vi "LIN_HoldEOL.vi"(5 "log?":bool, 7 "NAD":u8 format="%.0x", 8 "Error In":errorcluster caption="错误输入", 10 "exit":refnum<vi>, 11 "LIN Device":T1={"Master Frame(3C)"="MasterReq\nSPA3414_ConfigurationsCMAGeely_CEMCALYPSOSDB34XX0Cfg_LIN3_190709_", "Slave Frame(3D)"="SlaveResp\nSPA3414_ConfigurationsCMAGeely_CEMCALYPSOSDB34XX0Cfg_LIN3_190709_", "Request Schedule"="CEMLIN3DiagRequestSchedule\nSPA3414_ConfigurationsCMAGeely_CEMCALYPSOSDB34XX0Cfg_LIN3_190709_", "Response Schedule"="CEMLIN3DiagResponseSchedule\nSPA3414_ConfigurationsCMAGeely_CEMCALYPSOSDB34XX0Cfg_LIN3_190709_", "Frame Write SCU"="", "Frame Read SCU"="", "LIN Name"=""}) -> (0 "error IO":errorcluster)   [LabVIEW 2018]
uses:
  Crl/LIN_DataType.ctl
  user VI's/LIN/LIN Device.ctl
panel:
  in  "y":u32=3000
  out "LIN Device":T1={"Master Frame(3C)"="MasterReq\nSPA3414_ConfigurationsCMAGeely_CEMCALYPSOSDB34XX0Cfg_LIN3_190709_", "Slave Frame(3D)"="SlaveResp\nSPA3414_ConfigurationsCMAGeely_CEMCALYPSOSDB34XX0Cfg_LIN3_190709_", "Request Schedule"="CEMLIN3DiagRequestSchedule\nSPA3414_ConfigurationsCMAGeely_CEMCALYPSOSDB34XX0Cfg_LIN3_190709_", "Response Schedule"="CEMLIN3DiagResponseSchedule\nSPA3414_ConfigurationsCMAGeely_CEMCALYPSOSDB34XX0Cfg_LIN3_190709_", "Frame Write SCU"="", "Frame Read SCU"="", "LIN Name"=""}
  in  "Data":T2=[{"send?"=TRUE, "payload"=[2, 16, 3, 255, 255, 255, 255], "Delays"=0, "Note"="", "mult?"=FALSE, "Seq"=0}] {"payload" format="%02x"}
  # "ms"
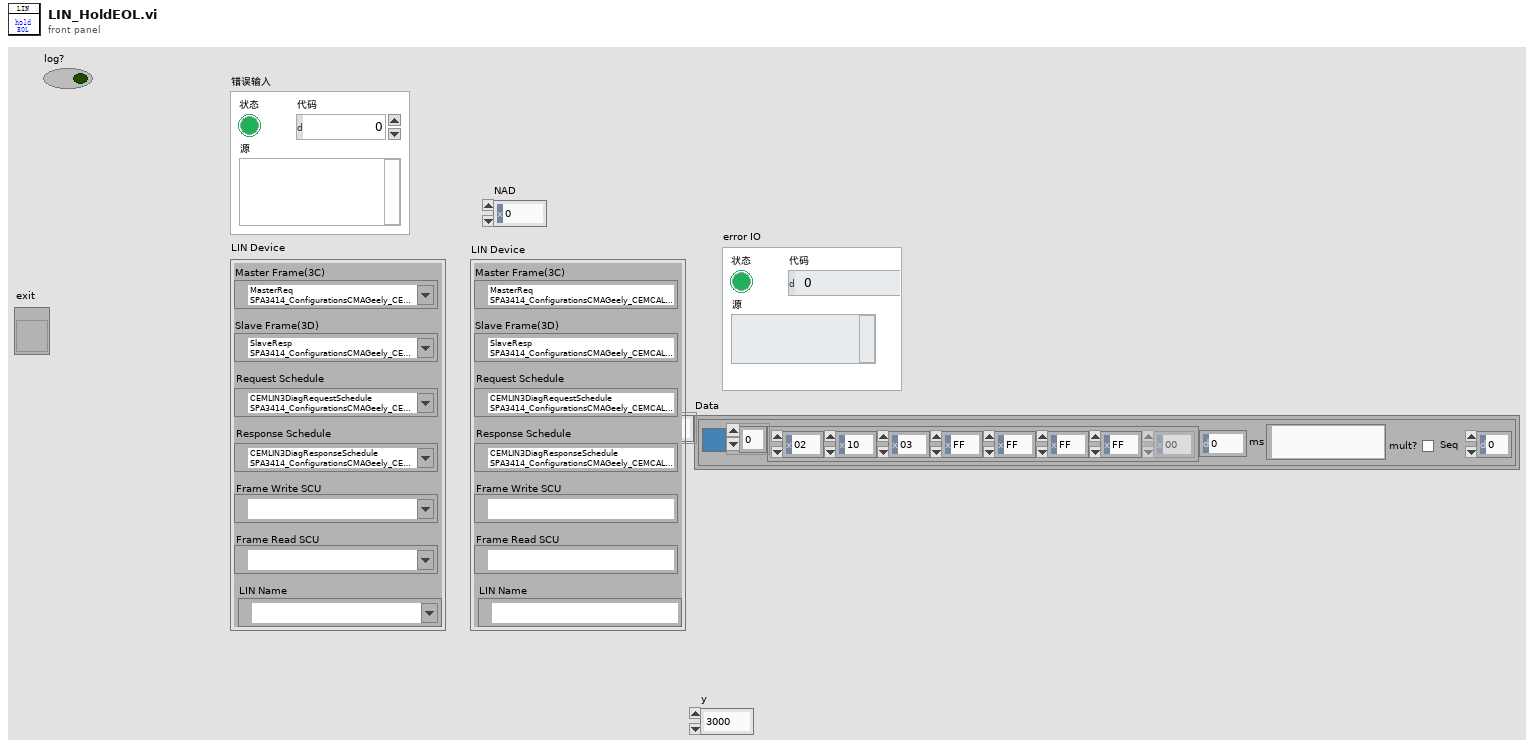
[diagram p1: front panel]
types:
  T1 = typedef "LIN Device.ctl" = cluster{"Master Frame(3C)":refnum<k21>, "Slave Frame(3D)":refnum<k21>, "Request Schedule":refnum<k21>, "Response Schedule":refnum<k21>, "Frame Write SCU":refnum<k21>, "Frame Read SCU":refnum<k21>, "LIN Name":refnum<k21>}
  T2 = typedef "LIN_DataType.ctl" = cluster{"send?":bool, "payload":u8[], "Delays":u32, "Note":string, "mult?":bool, "Seq":i32}[]
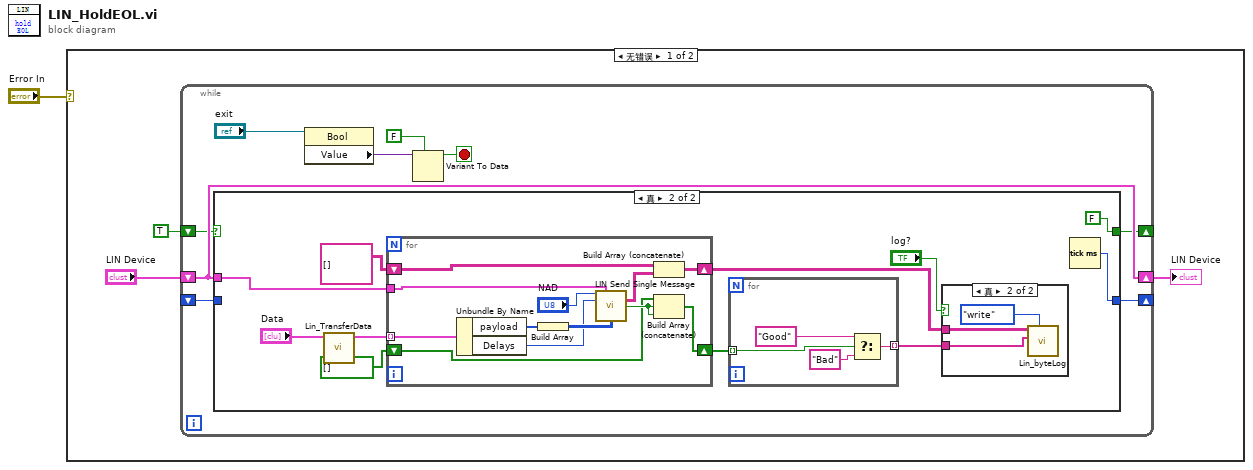
[diagram p0: block diagram]
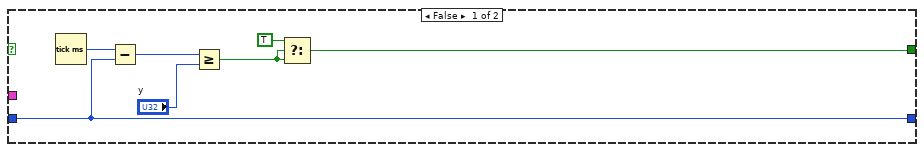
[diagram p2: hidden frame]
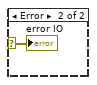
[diagram p4: hidden frame]
diagram:
  n1 = case shown="无错误" "Error In" {
    selector: "Error In" -> [_ w51]
    frame No Error {
      n2 = while {
        shift-right: [w13] -> w3
        shift-left: "LIN Device" -> [w13]
        shift-right: [w10] -> _
        shift-left: _ -> [w9]
        shift-right: [w11] -> _
        shift-left: TRUE -> [w12]
        stop <- w5 stop-if-true
        n3 = case shown="真" w12 {
          tunnel: w13 -> [_ w31]
          tunnel: w9 -> [w14 _]
          tunnel: [w18 FALSE] -> w11
          tunnel: [w14 w28] -> w10
          frame False {
            n4 = Tick Count (ms)() -> (millisecond timer value=w15:u32)
            n5 = Subtract(x=w15, y=w14) -> (x-y=w19:u32)
            n6 = Greater Or Equal?(x=w19, y="y") -> (x >= y?=w16:bool)
            n7 = Select(t=TRUE, s=w16, f=w16) -> (s? t:f=w18:bool)
          }
          frame True {
            n8 = call "Lin_TransferData.vi"("Data"="Data") -> ("Data"=w30:T2)  [unwired: 10 in]
            n9 = for {
              tunnel: w30 -> [w50] mode=indexing
              tunnel: w31 -> [w47]
              shift-right: [w43] -> w24
              shift-left: string[][] [] -> [w45]
              shift-right: [w42] -> w23
              shift-left: bool[] [] ("数组") -> [w40]
              n10 = Unbundle By Name(w50) -> ("payload"=w49:u8[], "Delays"=w46:u32)
              n11 = Build Array(w49) -> (w48:u8[][])
              n12 = call "LIN Send Single Message.vi"("NAD"="NAD", "LIN Device"=w47, "Msg Wait T"=w46, "Tx Msg"=w48) -> ("TxRx Data"=w44:string[][], "Response Good?"=w41:bool)  [unwired: 6 in, 4 out]
              n13 = Build Array (concatenate)(w45, w44) -> (w43:string[][])
              n14 = Build Array (concatenate)(w40, w41, w41) -> (w42:bool[])
            }
            n15 = for {
              tunnel: [w36] -> w25 mode=indexing
              tunnel: w23 -> [w35] mode=indexing
              n16 = Select(t="Good", s=w35, f="Bad") -> (s? t:f=w36:string)
            }
            n17 = case shown="真" "log?" {
              tunnel: w25 -> [_ w34]
              tunnel: w24 -> [_ w32]
              frame False {
              }
              frame True {
                n18 = call "Lin_byteLog.vi"("r/w"=enum16{"read", "write"}."write", "RespGood?"=w34, "TxRx Data"=w32) -> ()  [unwired: 8 in, 1 out]
              }
            }
            n19 = Tick Count (ms)() -> (millisecond timer value=w28:u32)
          }
        }
        n20 = property class="Bool"(reference="exit") -> ("Value"=w7:variant)  [unwired: 1 in, 2 out]
        n21 = Variant To Data(type=FALSE, Variant=w7) -> (data=w5:bool)  [unwired: 1 in, 1 out]
      }
      "LIN Device" <- w3
    }
    frame Error {
      "error IO" <- w51
    }
  }
